vi "Main.vi"(8 "error in":errorcluster, 11 "Network End Point in":refnum<class "Network End Point.lvclass">) -> (0 "error out":errorcluster, 3 "Network End Point out":refnum<class "Network End Point.lvclass">)   [LabVIEW 2020, in "Network End Point.lvclass"]
doc: "The Queued Message Handler of a Worker."
uses:
  Network End Point.lvclass
  C:/Program Files (x86)/National Instruments/LabVIEW 2020/vi.lib/addons/_Workers/Library/Classes/Worker/Worker.lvclass
  Network End Point.lvclass/Network End Point.ctl
  Initialization Data.ctl
  <vilib>/addons/_Workers/Library/Classes/Message Queue/Message Queue.lvclass
  <vilib>/addons/_Workers/Library/Classes/Message/Enqueue Message to Queue.vi
  TCP Receive/TCP Receive.lvclass
  TCP Send/TCP Send.lvclass
  <vilib>/addons/_Workers/Library/Classes/EHL/EHL.lvclass
  <vilib>/addons/_Workers/Library/Classes/Worker/Worker.lvclass
  <vilib>/addons/_Workers/Library/Classes/Error Handler/Error Handler.lvclass
  <vilib>/addons/_Workers/Library/Classes/Message/Message.lvclass
  C:/Program Files (x86)/National Instruments/LabVIEW 2020/vi.lib/addons/_Workers/Library/Classes/Worker User/Worker User.lvclass
  C:/Program Files (x86)/National Instruments/LabVIEW 2020/vi.lib/addons/_Workers/Library/Classes/Workers Object/Workers Object.lvclass
  C:/Users/TestAdmin/git/TCP-Workers/Workers/Network End Point/Network End Point.lvclass
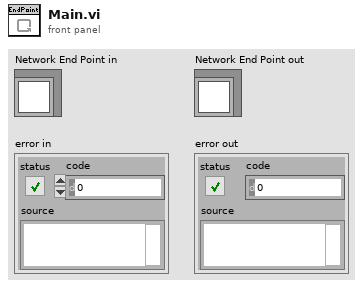
[diagram p1: front panel]
types:
  T1 = typedef "Network End Point.lvclass/Initialization Data.ctl" = cluster{"String":string, "Client":string, "connection ID":refnum<k5>, "Caller":refnum<class "Message Queue.lvclass">}
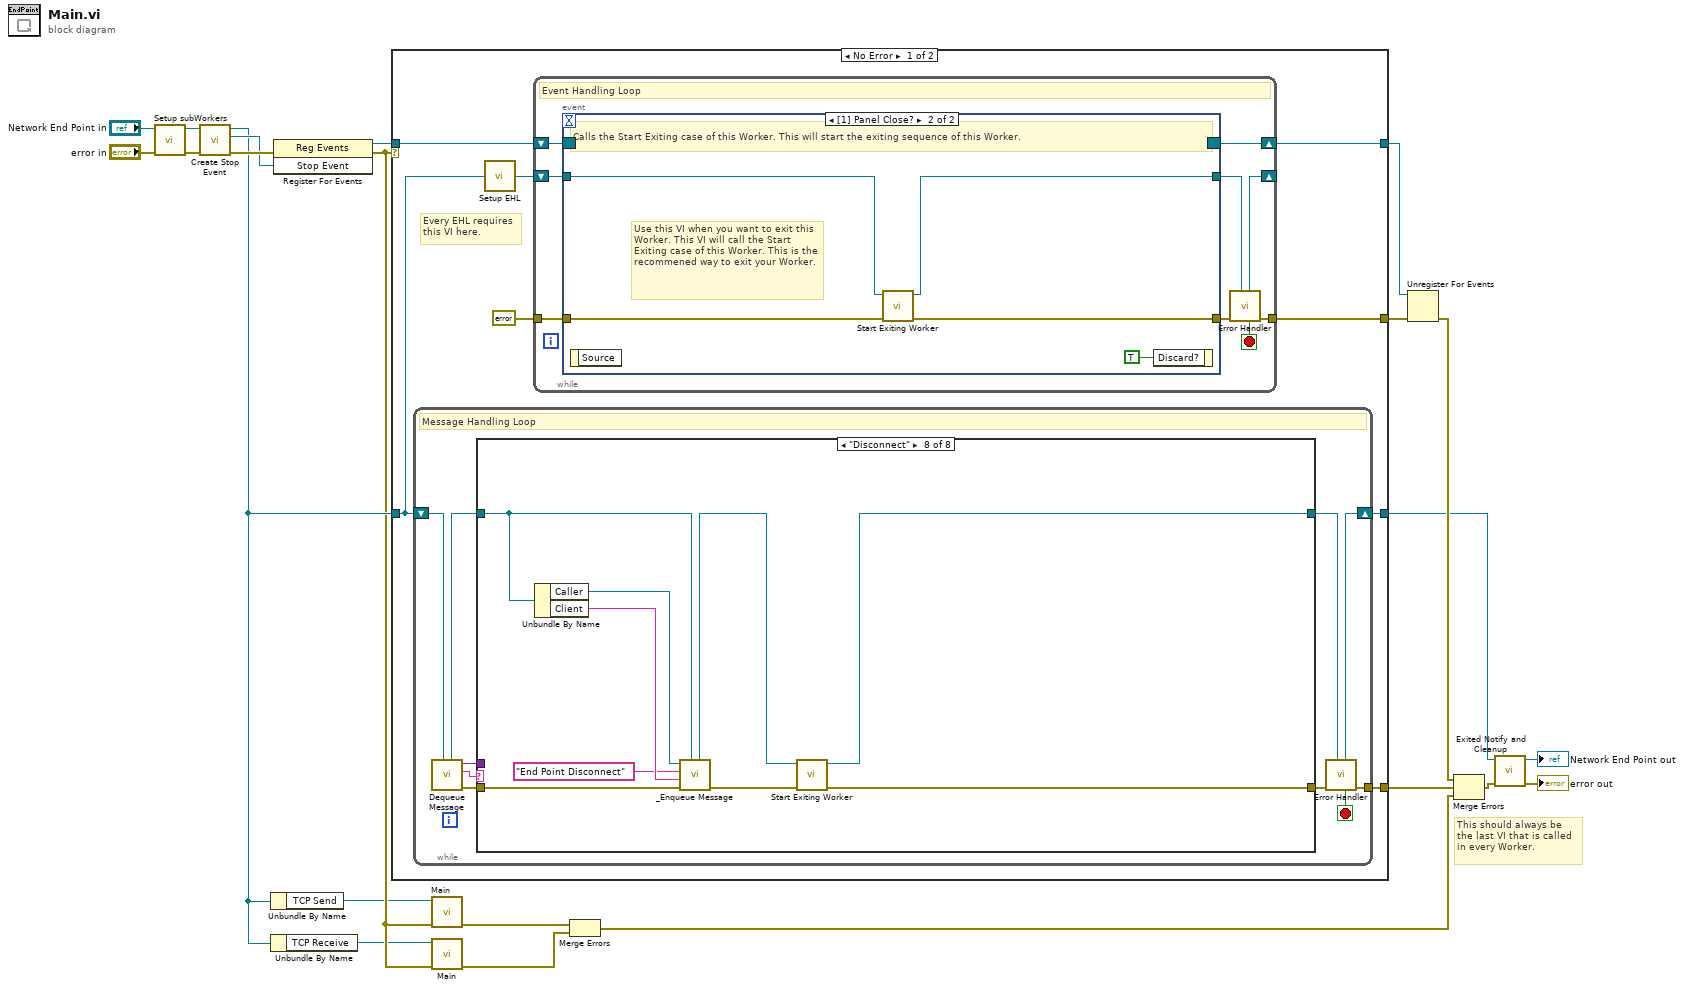
[diagram p0: block diagram]
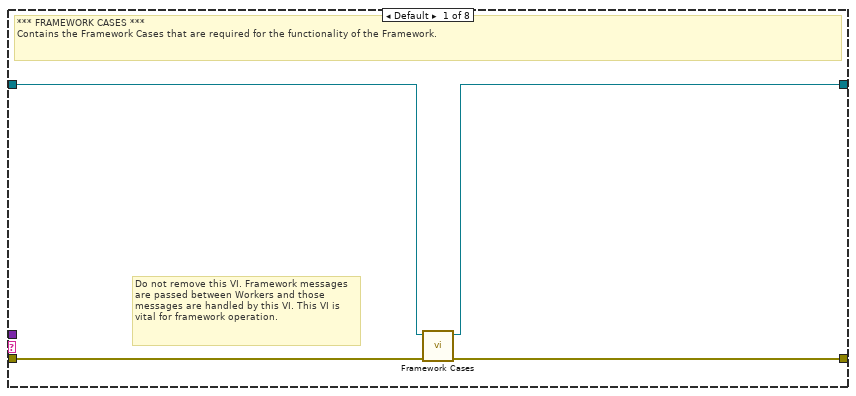
[diagram p2: hidden frame]
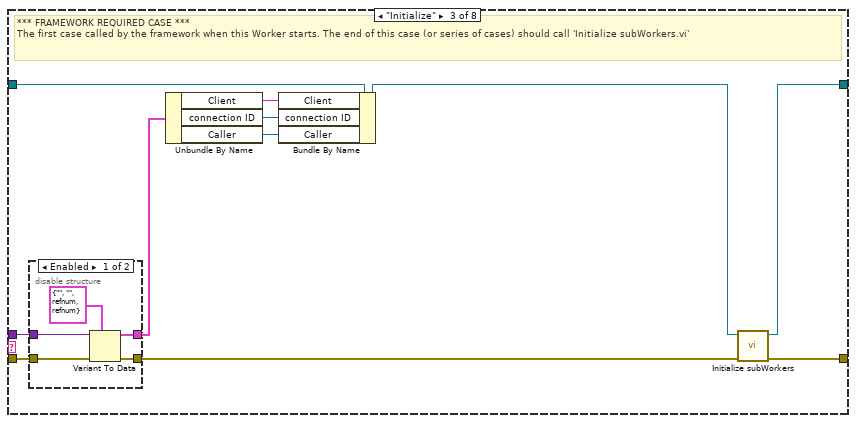
[diagram p4: hidden frame]
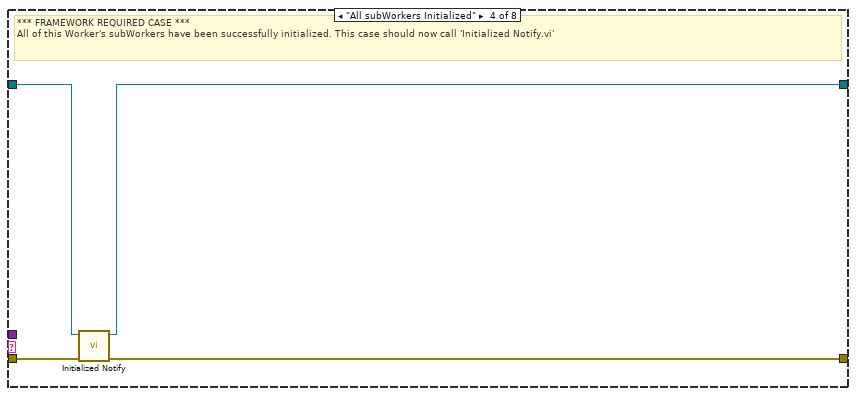
[diagram p6: hidden frame]
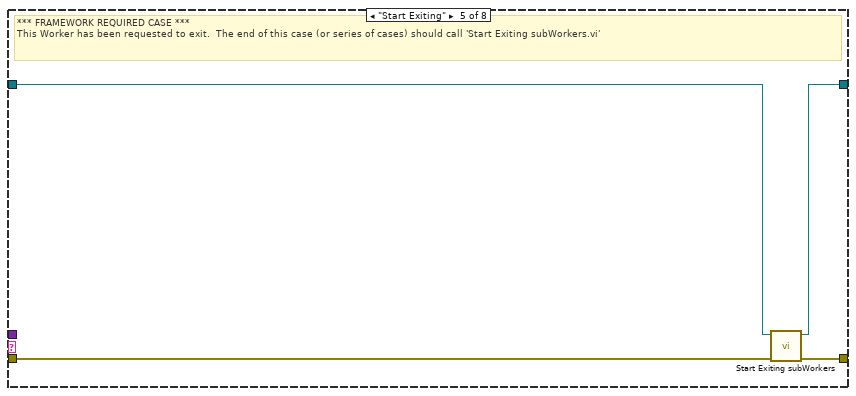
[diagram p7: hidden frame]
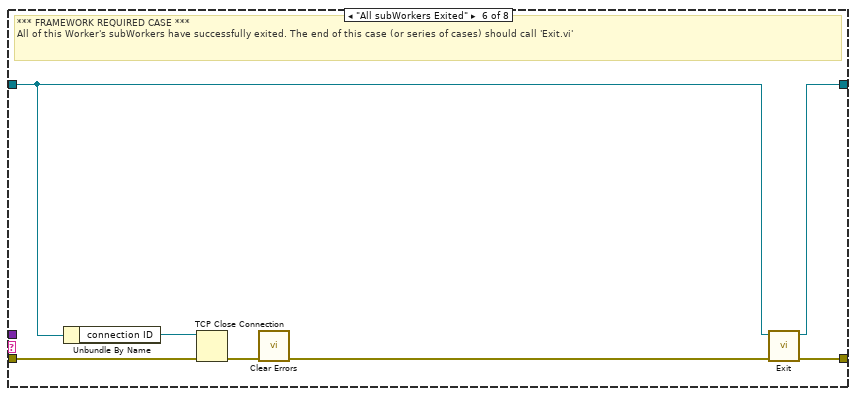
[diagram p8: hidden frame]
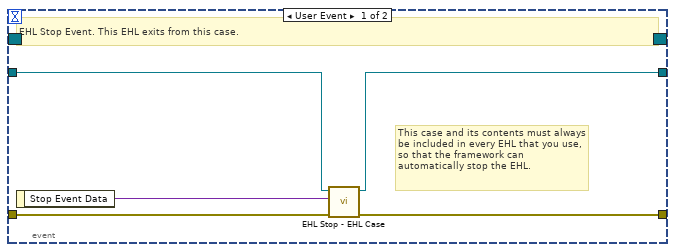
[diagram p10: hidden frame]
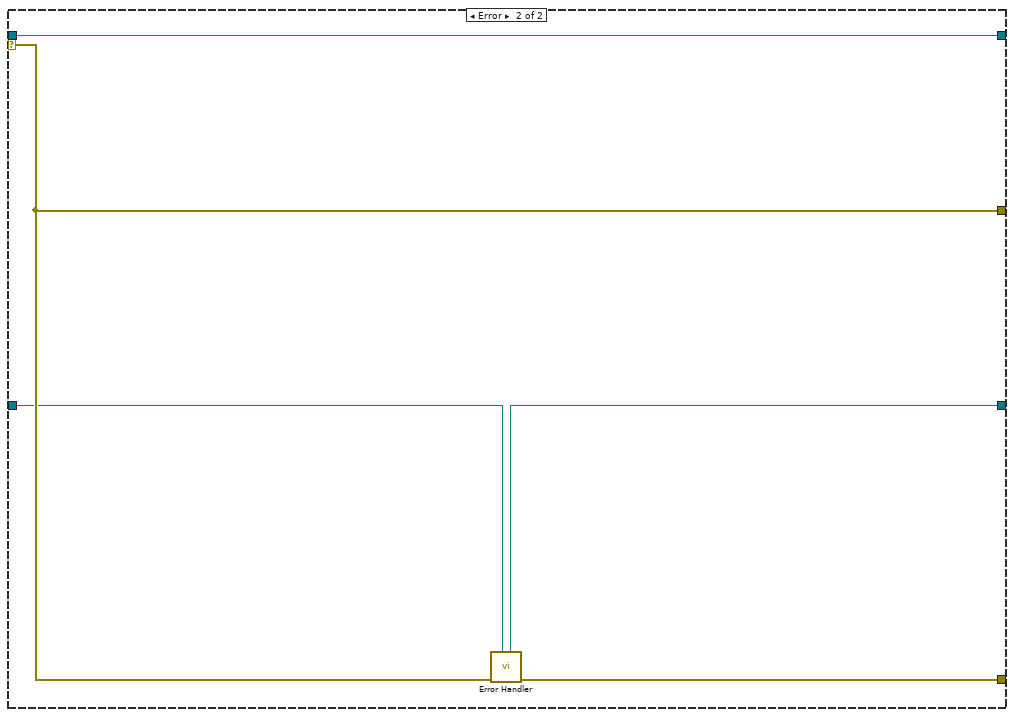
[diagram p11: hidden frame]
diagram:
  # "This should always be the last VI that is called in every Worker."
  n1 = call "Setup subWorkers.vi"("error in"="error in", "Network End Point in"="Network End Point in") -> ("error out"=w8:errorcluster, "Network End Point out"=w6:refnum<class "Network End Point.lvclass">)  [unwired: 8 in]
  n2 = call <vilib>:"Create Stop Event.vi"("error in"=w8, "Worker"=w6) -> ("error out"=w17:errorcluster, "Stop Event"=w14:refnum<user-event>, "Worker out"=w11:refnum<class "Network End Point.lvclass">)  [unwired: 7 in]
  n3 = Unbundle By Name(w11) -> ("TCP Send"=w3:refnum<class "TCP Send.lvclass">)
  n4 = Unbundle By Name(w11) -> ("TCP Receive"=w1:refnum<class "TCP Receive.lvclass">)
  n5 = register-events(error in=w17, w14) -> (reference out=w16:refnum<event-registration>, error out=w9:errorcluster)  [unwired: 1 in]
  n6 = case shown="No Error" w9 {
    tunnel: w11 -> [w25 w110]
    tunnel: [w23 w111] -> w15
    tunnel: w16 -> [w30 w112]
    tunnel: [w27 w113] -> w21
    tunnel: [w29 w112] -> w20
    tunnel: [w24 w109] -> w18
    selector: w9 -> [_ w113]
    frame No Error {
      # "Every EHL requires\nthis VI here."
      n7 = while {
        shift-right: [w38] -> w24
        shift-left: w25 -> [w40]
        tunnel: [w39] -> w23
        stop <- w32 stop-if-true
        # "Message Handling Loop"
        n8 = call <vilib>:"Dequeue Message.vi"("Worker"=w40) -> ("error out"=w37:errorcluster, "Case out"=w31:string, "Data out"=w33:variant, "Worker out"=w35:refnum<class "Network End Point.lvclass">)  [unwired: 6 in, 1 out]
        n9 = case "WORKERS MHL Case Structure (DO NOT CHANGE LABEL NAME)" shown="\"Disconnect\"" w31 {
          tunnel: w37 -> [w44 w45 w55 w67 w68 w74 w79 w89]
          tunnel: [w43 w45 w57 w66 w71 w78 w79 w83] -> w36
          tunnel: w35 -> [w42 w46 w54 w64 w69 w72 w80 w88]
          tunnel: [w41 w46 w56 w65 w70 w77 w80 w81] -> w34
          tunnel: w33 -> [_ _ w52 _ _ _ _ _]
          frame Default {
            # "Do not remove this VI. Framework messages are passed between Workers and those messages are handled by this VI. This VI is vital for framework operation."
            # "*** FRAMEWORK CASES ***\nContains the Framework Cases that are required for the functionality of the Framework."
            n10 = call <vilib>:"Framework Cases.vi"("error in"=w44, "Worker"=w42) -> ("error out"=w43:errorcluster, "Worker out"=w41:refnum<class "Network End Point.lvclass">)  [unwired: 8 in]
          }
          frame "------ FRAMEWORK REQUIRED CASES ------" {
            # "Start of Framework Required Cases"
          }
          frame "Initialize" {
            # "*** FRAMEWORK REQUIRED CASE ***\nThe first case called by the framework when this Worker starts. The end of this case (or series of cases) should call 'Initialize subWorkers.vi'"
            n11 = disable-structure shown="Enabled" {
              disable-tunnel: w55 -> [w62 w63]
              disable-tunnel: [w61 w63] -> w53
              disable-tunnel: w52 -> [w60 _]
              disable-tunnel: [w58 _] -> w50
              frame Enabled {
                n12 = Variant To Data(error in=w62, type=T1 {"String"="", "Client"="", "connection ID"=refnum, "Caller"=refnum} ("Initialization Data"), Variant=w60) -> (data=w58:T1, error out=w61:errorcluster)
              }
              frame Disabled {
              }
            }
            n13 = Unbundle By Name(w50) -> ("Client"=w49:string, "connection ID"=w48:refnum<k5>, "Caller"=w47:refnum<class "Message Queue.lvclass">)
            n14 = Bundle By Name(cluster=w54, "Client"=w49, "connection ID"=w48, "Caller"=w47) -> (w51:refnum<class "Network End Point.lvclass">)
            n15 = call <vilib>:"Initialize subWorkers.vi"("error in"=w53, "Worker"=w51) -> ("error out"=w57:errorcluster, "dup Worker out"=w56:refnum<class "Network End Point.lvclass">)  [unwired: 8 in]
          }
          frame "All subWorkers Initialized" {
            # "*** FRAMEWORK REQUIRED CASE ***\nAll of this Worker's subWorkers have been successfully initialized. This case should now call 'Initialized Notify.vi'"
            n16 = call <vilib>:"Initialized Notify.vi"("error in"=w67, "Worker"=w64) -> ("error out"=w66:errorcluster, "dup Worker out"=w65:refnum<class "Network End Point.lvclass">)  [unwired: 8 in]
          }
          frame "Start Exiting" {
            # "*** FRAMEWORK REQUIRED CASE ***\nThis Worker has been requested to exit.  The end of this case (or series of cases) should call 'Start Exiting subWorkers.vi'"
            n17 = call <vilib>:"Start Exiting subWorkers.vi"("error_in"=w68, "Worker"=w69) -> ("error out"=w71:errorcluster, "dup Worker out"=w70:refnum<class "Network End Point.lvclass">)  [unwired: 8 in]
          }
          frame "All subWorkers Exited" {
            # "*** FRAMEWORK REQUIRED CASE ***\nAll of this Worker's subWorkers have successfully exited. The end of this case (or series of cases) should call 'Exit.vi'"
            n18 = Unbundle By Name(w72) -> ("connection ID"=w76:refnum<k5>)
            n19 = TCP Close Connection(connection ID=w76, error in (no error)=w74) -> (error out=w75:errorcluster)  [unwired: 1 in, 1 out]
            n20 = call <vilib>:"Clear Errors.vi"("error in (no error)"=w75) -> ("error out"=w73:errorcluster)  [unwired: 5 in, 1 out]
            n21 = call <vilib>:"Exit.vi"("error_in"=w73, "Worker"=w72) -> ("error out"=w78:errorcluster, "dup Worker out"=w77:refnum<class "Network End Point.lvclass">)  [unwired: 8 in]
          }
          frame "-----------------------------------------------" {
            # "End of Framework Required Cases"
          }
          frame "Disconnect" {
            n22 = Unbundle By Name(w88) -> ("Caller"=w87:refnum<class "Message Queue.lvclass">, "Client"=w86:string)
            n23 = call-poly <vilib>:"_Enqueue Message.vi"("Worker"=w88, "error in"=w89, "Data"=w86, "Case Label"="End Point Disconnect", "Message Queue"=w87) -> ("error out"=w84:errorcluster, "dup Worker out"=w82:refnum<class "Network End Point.lvclass">)  [unwired: 4 in, 1 out]
            n24 = call <vilib>:"Start Exiting Worker.vi"("error in"=w84, "Worker"=w82) -> ("error out"=w83:errorcluster, "dup Worker out"=w81:refnum<class "Network End Point.lvclass">)  [unwired: 8 in]
          }
        }
        n25 = call <vilib>:"Error Handler.vi"("Worker"=w34, "error_in"=w36) -> ("error out"=w39:errorcluster, "Stop Loop"=w32:bool, "Worker out"=w38:refnum<class "Network End Point.lvclass">)  [unwired: 7 in]
      }
      n26 = call <vilib>:"Setup EHL.vi"("Worker"=w25) -> ("Worker out"=w26:refnum<class "Network End Point.lvclass">)  [unwired: 14 in]
      n27 = while "Event Handling Loop" {
        shift-right: [w98] -> w29
        shift-left: w30 -> [w97]
        tunnel: [w93] -> w27
        tunnel: errorcluster {"status"=FALSE, "code"=0, "source"=""} ("error constant") -> [w95]
        shift-right: [w91] -> _
        shift-left: w26 -> [w96]
        stop <- w90 stop-if-true
        # "Event Handling Loop"
        n28 = event shown="[1] Panel Close?" {
          selector: w97 -> [_ _]
          dyn-events: [_ _] -> w98
          timeout: _ -> [_ _]
          tunnel: [w102 w107] -> w94
          tunnel: w95 -> [w103 w106]
          tunnel: w96 -> [w101 w105]
          tunnel: [w100 w104] -> w92
          event User Event {
            # "This case and its contents must always be included in every EHL that you use, so that the framework can automatically stop the EHL."
            # "EHL Stop Event. This EHL exits from this case."
            n29 = event-data() -> ("Stop Event Data"=w99:variant)  [unwired: 1 in]
            n30 = call <vilib>:"EHL Stop - EHL Case.vi"("error in"=w103, "Stop Event Data"=w99, "Worker"=w101) -> ("error out"=w102:errorcluster, "Worker out"=w100:refnum<class "Network End Point.lvclass">)  [unwired: 7 in]
          }
          event Panel Close? {
            # "Use this VI when you want to exit this Worker. This VI will call the Start Exiting case of this Worker. This is the recommened way to exit your Worker."
            # "Calls the Start Exiting case of this Worker. This will start the exiting sequence of this Worker."
            n31 = event-data() -> ()  [unwired: 1 in, 1 out]
            n32 = call <vilib>:"Start Exiting Worker.vi"("error in"=w106, "Worker"=w105) -> ("error out"=w107:errorcluster, "dup Worker out"=w104:refnum<class "Network End Point.lvclass">)  [unwired: 8 in]
            n33 = event-data ("Event Filter Node")("Discard?"=TRUE) -> ()  [unwired: 1 in, 1 out]
          }
        }
        n34 = call <vilib>:"Error Handler.vi"("Worker"=w92, "error_in"=w94) -> ("error out"=w93:errorcluster, "Stop Loop"=w90:bool, "Worker out"=w91:refnum<class "Network End Point.lvclass">)  [unwired: 7 in]
      }
    }
    frame Error {
      n35 = call <vilib>:"Error Handler.vi"("Worker"=w110, "error_in"=w113) -> ("error out"=w111:errorcluster, "Worker out"=w109:refnum<class "Network End Point.lvclass">)  [unwired: 7 in, 1 out]
    }
  }
  n36 = call-dynamic "Main.vi"("error in"=w9, "TCP Send in"=w3) -> ("error out"=w5:errorcluster)  [unwired: 8 in, 1 out]
  n37 = call-dynamic "Main.vi"("error in"=w9, "TCP Receive in"=w1) -> ("error out"=w2:errorcluster)  [unwired: 8 in, 1 out]
  n38 = Merge Errors(w5, w2) -> (w4:errorcluster)
  n39 = Unregister For Events(event registration refnum=w20, error in=w21) -> (error out=w22:errorcluster)
  n40 = Merge Errors(w22, w15, w4) -> (w19:errorcluster)
  n41 = call <vilib>:"Exited Notify and Cleanup.vi"("error_in"=w19, "Worker"=w18) -> ("error out"=→"error out":errorcluster, "dup Worker out"=→"Network End Point out":refnum<class "Network End Point.lvclass">)  [unwired: 8 in]
